vi "LJstreamUD data file write.vi"(0 "Starting #":u32, 2 "Time":dbl format="%.2f", 4 "Scan Rate":dbl=50.0 format="%.2f", 5 "Data File Prefix":string="data", 6 "Channel Config":T1={"# Channels"=4, "+Ch"=["0", "1", "2", "3", "4", "5", "6", "7"], "-Ch (U3)"=["31", "31", "31", "31", "31", "31", "31", "31"], "Ranges (UE9)"=[0, 0, 0, 0, 0, 0, 0, 0], "Scaling Equation"=["y=v0", "y=v1", "y=v2", "y=v3", "y=v4", "y=v5", "y=v6", "y=v7"]} {"Ranges (UE9)" items=["LJ_rgBIP5V", "LJ_rgUNI5V", "LJ_rgUNI2P5V", "LJ_rgUNI1P25V", "LJ_rgUNIP625V"]}, 7 "Write To File":bool, 8 "max file size (bytes)":i32=100000000, 9 "Scaled Data":dbl[][](array[numeric]) format="%.3f", 10 "Voltages":dbl[][](array[numeric]) format="%.3f", 11 "Current Data File In":path) -> (1 "Data File #":u32, 3 "Current Data File Out":path)   [LabVIEW 2021]
uses:
  LJstreamUD globals.vi
panel:
  out "ms":u32
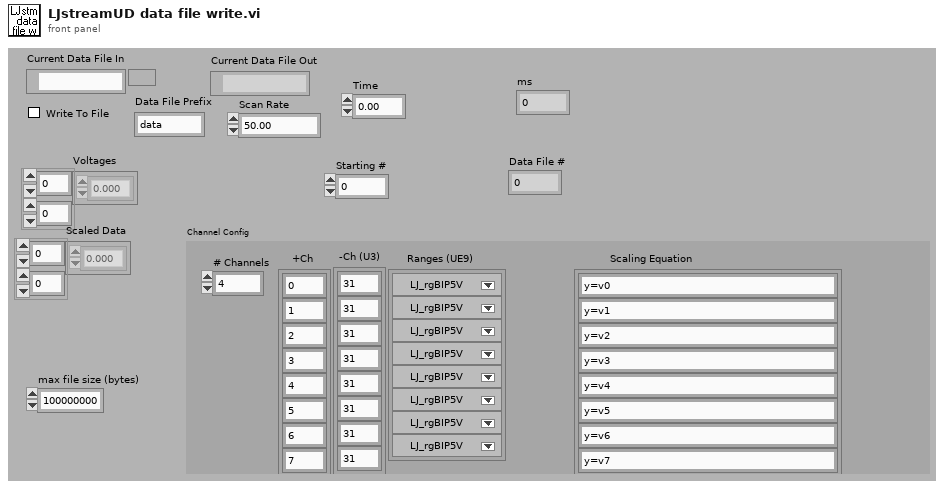
[diagram p1: front panel]
types:
  T1 = cluster{"# Channels":i32, "+Ch":string[], "-Ch (U3)":string[], "Ranges (UE9)":u16[], "Scaling Equation":string[]}
  T2 = enum16{"open", "open or create", "create or replace", "create", "open (read only)"}
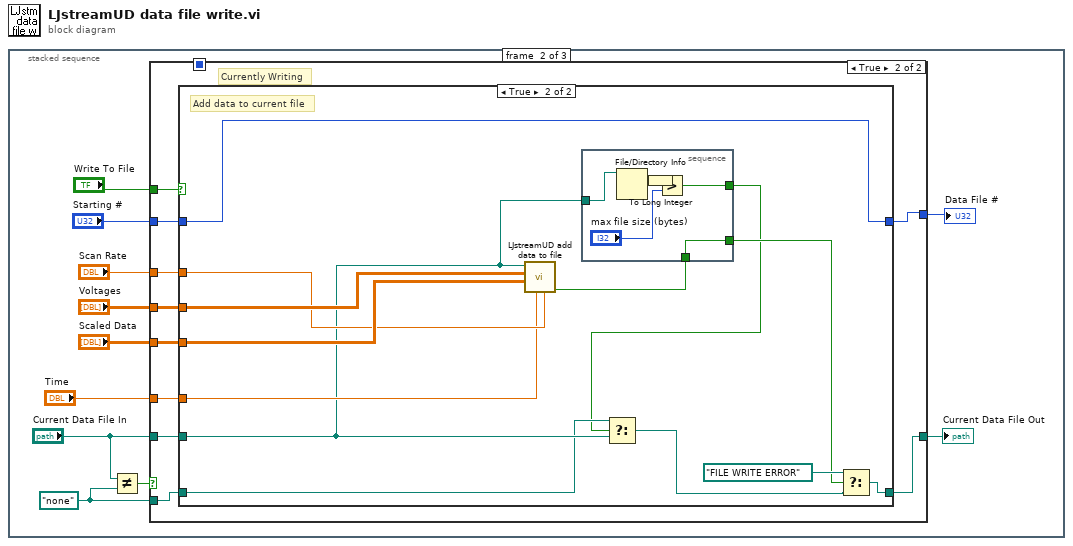
[diagram p0: block diagram]
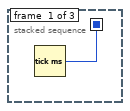
[diagram p2: hidden frame]
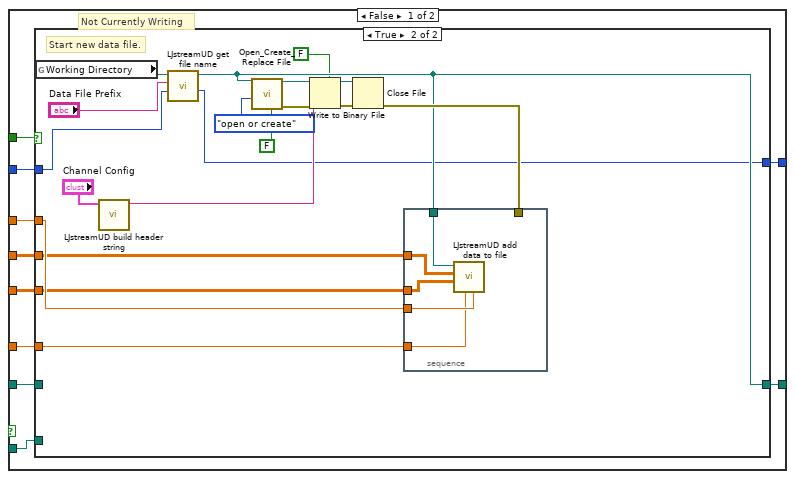
[diagram p3: hidden frame]
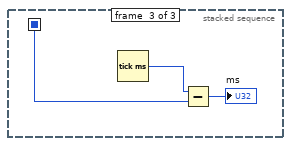
[diagram p6: hidden frame]
diagram:
  n1 = stacked-sequence {
    seq-local: [w1 _ _] -> [_ _ w81]
    frame #0 {
      n2 = Tick Count (ms)() -> (millisecond timer value=w1:u32)
    }
    frame #1 {
      w8 = path "none" ("y")
      n3 = Not Equal?(x="Current Data File In", y=w8) -> (x != y?=w12:bool)
      n4 = case shown="True" w12 {
        tunnel: "Current Data File In" -> [w22 w58]
        tunnel: "Write To File" -> [w20 w57]
        tunnel: [w21 w55] -> w9
        tunnel: w8 -> [w19 w56]
        tunnel: "Voltages" -> [w16 w54]
        tunnel: "Scaled Data" -> [w15 w53]
        tunnel: "Scan Rate" -> [w18 w52]
        tunnel: "Time" -> [w17 w51]
        tunnel: "Starting #" -> [w14 w50]
        tunnel: [w13 w49] -> w2
        frame False {
          # "Not Currently Writing"
          n5 = case shown="True" w20 {
            tunnel: w22 -> [_ _]
            tunnel: [w24 w34] -> w21
            tunnel: w19 -> [w24 _]
            tunnel: w18 -> [_ w33]
            tunnel: w17 -> [_ w32]
            tunnel: w16 -> [_ w31]
            tunnel: w15 -> [_ w30]
            tunnel: w14 -> [w23 w27]
            tunnel: [w23 w26] -> w13
            frame False {
              # "Do nothing"
            }
            frame True {
              # "Start new data file."
              n6 = global read "LJstreamUD globals.vi" "Working Directory"() -> (w29:path)
              n7 = call "LJstreamUD build header string.vi"("Channel Config"="Channel Config") -> ("Header String"=w36:string)  [unwired: 10 in]
              n8 = call "LJstreamUD get file name.vi"("Starting #"=w27, "Data File Prefix"="Data File Prefix", "Working Directory"=w29) -> ("Data File #"=w26:u32, "Data File Path"=w34:path)  [unwired: 7 in]
              n9 = call <vilib>:"Open_Create_Replace File.vi"("advisory dialog? (display:T)"=FALSE, "function (open:0)"=T2."open or create", "file path"=w34) -> ("error out"=w40:errorcluster, "refnum"=w39:refnum<file>)  [unwired: 5 in, 2 out]
              n10 = Write to Binary File(file (use dialog)=w39, data=w36, error in=w40, 5:FALSE ("prepend array or string size? (T)")) -> (refnum out=w37:refnum<file>, error out=w38:errorcluster)  [unwired: 2 in, 1 out]
              n11 = Close File(refnum=w37, error in=w38) -> (error out=w35:errorcluster)  [unwired: 1 out]
              n12 = stacked-sequence {
                tunnel: w35 -> [_]
                tunnel: w34 -> [w48]
                tunnel: w33 -> [w47]
                tunnel: w32 -> [w46]
                tunnel: w31 -> [w45]
                tunnel: w30 -> [w44]
                frame #0 {
                  n13 = call "LJstreamUD add data to file.vi"("Scan Rate"=w47, "Time"=w46, "Scaled Data"=w44, "Voltages"=w45, "file path"=w48) -> ()  [unwired: 6 in, 1 out]
                }
              }
            }
          }
        }
        frame True {
          # "Currently Writing"
          n14 = case shown="True" w57 {
            tunnel: w58 -> [_ w65]
            tunnel: [w60 w66] -> w55
            tunnel: w56 -> [w60 w63]
            tunnel: w54 -> [_ w72]
            tunnel: w53 -> [_ w71]
            tunnel: w52 -> [_ w70]
            tunnel: w51 -> [_ w69]
            tunnel: w50 -> [w59 w61]
            tunnel: [w59 w61] -> w49
            frame False {
              # "Stop writing to current data file."
            }
            frame True {
              # "Add data to current file"
              n15 = call "LJstreamUD add data to file.vi"("Scan Rate"=w70, "Time"=w69, "Scaled Data"=w71, "Voltages"=w72, "file path"=w65) -> ("error"=w68:bool)  [unwired: 6 in]
              n16 = stacked-sequence {
                tunnel: w68 -> [w79]
                tunnel: [w79] -> w67
                tunnel: w65 -> [w78]
                tunnel: [w76] -> w62
                frame #0 {
                  n17 = File/Directory Info(path=w78) -> (size=w74:i64)  [unwired: 1 in, 6 out]
                  n18 = To Long Integer(number=w74) -> (32bit integer=w77:i32)
                  n19 = Greater?(x=w77, y="max file size (bytes)") -> (0:w76:bool)
                }
              }
              n20 = Select(t=w63, s=w62, f=w65) -> (s? t:f=w64:path)
              n21 = Select(t=path "FILE WRITE ERROR", s=w67, f=w64) -> (s? t:f=w66:path)
            }
          }
        }
      }
      "Current Data File Out" <- w9
      "Data File #" <- w2
    }
    frame #2 {
      n22 = Tick Count (ms)() -> (millisecond timer value=w82:u32)
      n23 = Subtract(x=w82, y=w81) -> (x-y=→"ms":u32)
    }
  }
